vi "Fire Collapse Event.vi"(8 "error in (no error)":errorcluster, 10 "Collapsed":T1, 11 "GVIWebProcessorApp in":refnum<class "GVIWebProcessorApp.lvclass">) -> (0 "error out":errorcluster, 3 "GVIWebProcessorApp out":refnum<class "GVIWebProcessorApp.lvclass">)   [LabVIEW 2020, in "PicoG-Processor.lvlib" / "GVIWebProcessorApp.lvclass"]
uses:
  GVIWebProcessorApp.lvclass
  Set Collapsed UI Event.ctl
  GVIWebProcessorApp.lvclass/GVIWebProcessorApp.ctl
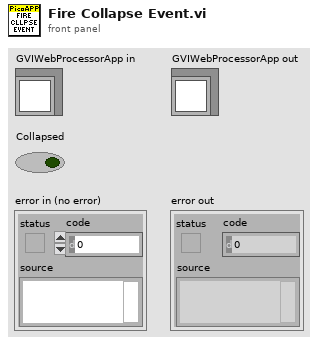
[diagram p1: front panel]
types:
  T1 = typedef "PicoG-Processor.lvlib/GVIWebProcessorApp.lvclass/Set Collapsed UI Event.ctl" = bool
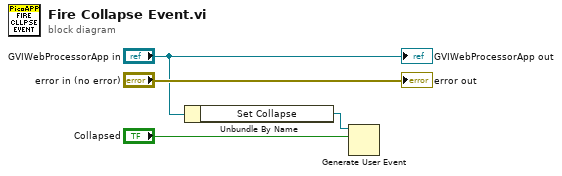
[diagram p0: block diagram]
diagram:
  n1 = Unbundle By Name("GVIWebProcessorApp in") -> ("Set Collapse"=w2:refnum<user-event>)
  n2 = Generate User Event(user event=w2, event data cluster="Collapsed") -> ()  [unwired: 2 in, 2 out]
  "error out" <- "error in (no error)"
  "GVIWebProcessorApp out" <- "GVIWebProcessorApp in"
